vi "Manueel_geautomatiseerd.vi"() -> ()   [LabVIEW 2019]
panel:
  out "Numeric 3":dbl
  in  "Boolean":bool
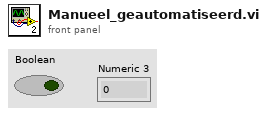
[diagram p1: front panel]
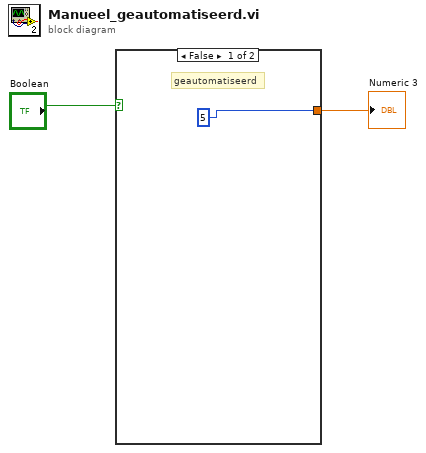
[diagram p0: block diagram]
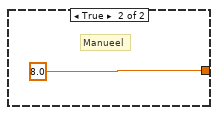
[diagram p2: hidden frame]
diagram:
  n1 = case shown="False" "Boolean" {
    tunnel: [5 8.0] -> w1
    frame False {
      # "geautomatiseerd"
    }
    frame True {
      # "Manueel"
    }
  }
  "Numeric 3" <- w1
